vi "DFS Data - Get Node.vi"(8 "Error In":errorcluster, 10 "Node Index":i32, 11 "DFS Data":T3) -> (0 "Error Out":errorcluster, 3 "DFS Node":T1)   [LabVIEW 2022 SP3]
doc: "<add documentation here>"
uses:
  DFS Data (cluster).ctl
  DFS Node (cluster).ctl
  DFS Child Node (cluster).ctl
panel:
  # "Development\nControls or indicators that are useful for development or testing, but which are not outputs of the VI."
  # "Input\nInputs to the VI"
  # "Output\nOutputs of the VI"
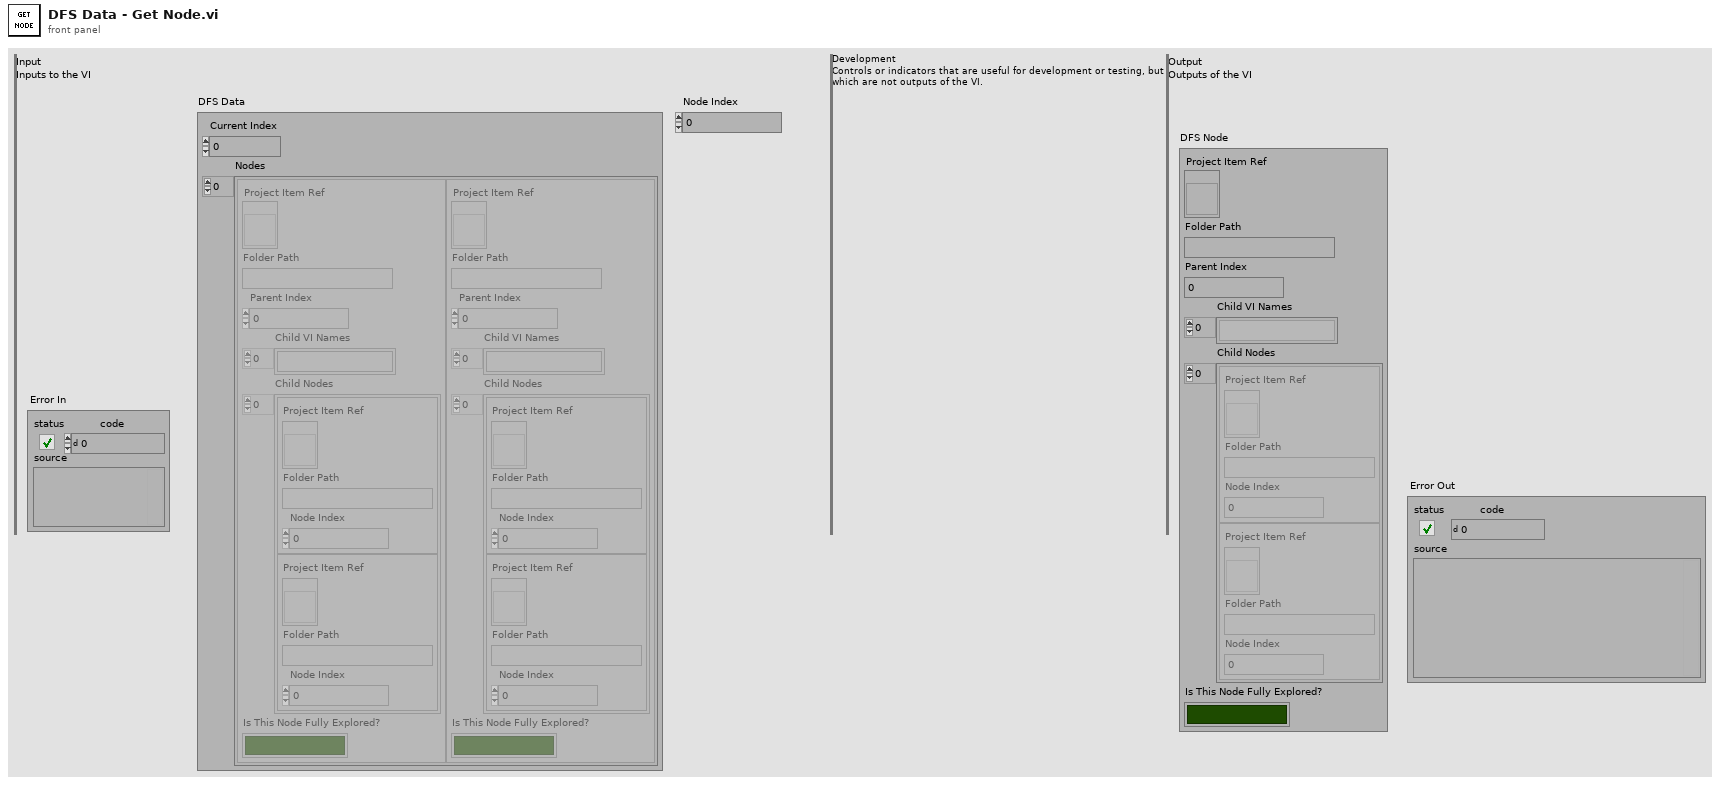
[diagram p1: front panel]
types:
  T1 = typedef "DFS Node (cluster).ctl" = cluster{"Project Item Ref":refnum<vi>, "Folder Path":string, "Parent Index":i32, "Child VI Names":string[], "Child Nodes":T2[], "Is This Node Fully Explored?":bool}
  T2 = typedef "DFS Child Node (cluster).ctl" = cluster{"Project Item Ref":refnum<vi>, "Folder Path":string, "Node Index":i32}
  T3 = typedef "DFS Data (cluster).ctl" = cluster{"Current Index":i32, "Nodes":T1[]}
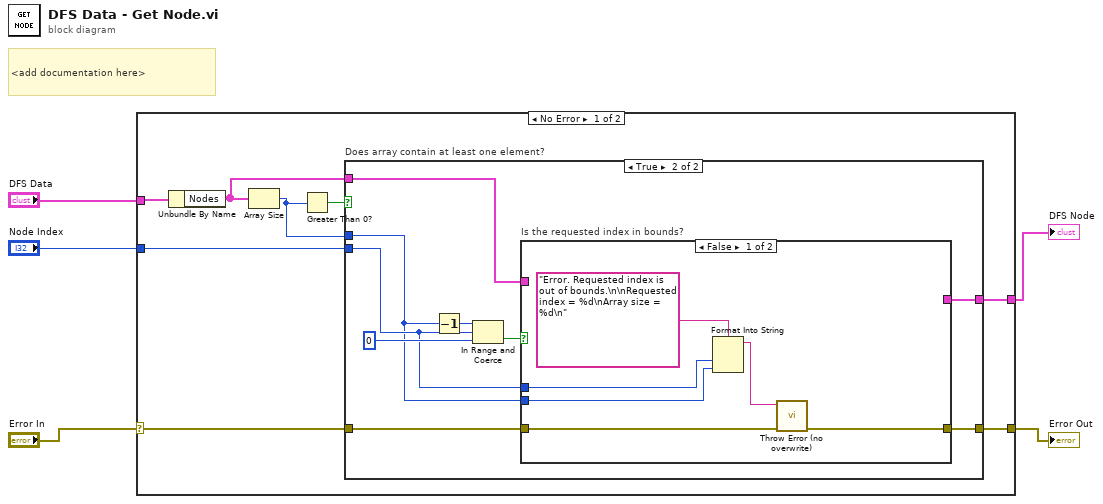
[diagram p0: block diagram]
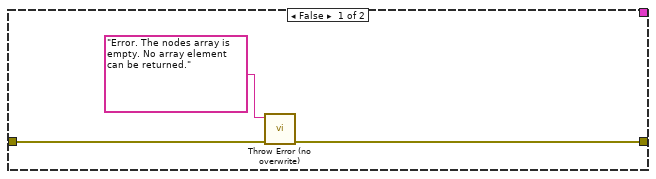
[diagram p2: hidden frame]
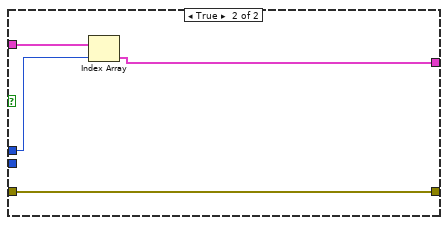
[diagram p3: hidden frame]
diagram:
  # "<add documentation here>"
  n1 = case shown="No Error" "Error In" {
    selector: "Error In" -> [w12 w36]
    tunnel: [w11 w36] -> w4
    tunnel: "Node Index" -> [w9 _]
    tunnel: "DFS Data" -> [w13 _]
    tunnel: [w6 _] -> w1
    frame No Error {
      n2 = Unbundle By Name(w13) -> ("Nodes"=w7:T1[])
      n3 = Array Size(array=w7) -> (size(s)=w8:i32)
      n4 = Greater Than 0?(x=w8) -> (x > 0?=w10:bool)
      n5 = case "Does array contain at least one element?" shown="True" w10 {
        tunnel: w12 -> [w16 w23]
        tunnel: [w15 w22] -> w11
        tunnel: w9 -> [_ w20]
        tunnel: w8 -> [_ w19]
        tunnel: w7 -> [_ w18]
        tunnel: [_ w17] -> w6
        frame False {
          n6 = call "Throw Error (no overwrite).vi"("error in"=w16, "Error Message"="Error. The nodes array is empty. No array element can be returned.") -> ("error out"=w15:errorcluster)  [unwired: 9 in]
        }
        frame True {
          n7 = Decrement(x=w19) -> (x-1=w24:i32)
          n8 = In Range and Coerce(upper limit=w24, x=w20, lower limit=0) -> (In Range?=w21:bool)  [unwired: 1 out]
          n9 = case "Is the requested index in bounds?" shown="False" w21 {
            tunnel: w23 -> [w31 w35]
            tunnel: [w30 w35] -> w22
            tunnel: w20 -> [w27 w33]
            tunnel: w19 -> [w26 _]
            tunnel: w18 -> [_ w34]
            tunnel: [_ w32] -> w17
            frame False {
              n10 = Format Into String(format string="Error. Requested index is out of bounds.\n\nRequested index = %d\nArray size = %d\n", w27, w26) -> (resulting string=w28:string)  [unwired: 2 in, 1 out]
              n11 = call "Throw Error (no overwrite).vi"("error in"=w31, "Error Message"=w28) -> ("error out"=w30:errorcluster)  [unwired: 9 in]
            }
            frame True {
              n12 = Index Array(array=w34, index=w33) -> (element=w32:T1)
            }
          }
        }
      }
    }
    frame Error {
    }
  }
  "Error Out" <- w4
  "DFS Node" <- w1
